vi "Image receiving and storage.vi"() -> ()   [LabVIEW 2009]
uses:
  <vilib>/vision/Image Controls.llb/IMAQ Image.ctl
panel:
  in  "A":bool=TRUE
  in  "¼v¹³Àx¦s¶s":bool
  in  "±i/¨C¬í":u32=30
  out "Àx¦s¸ô®|":path
  in  "connection in":string="dstp://192.168.1.100/image"
  in  "Äá¼v¾÷°±¤î¶s":bool
  out "«eÄá¼v¾÷":T1(plugin-control)
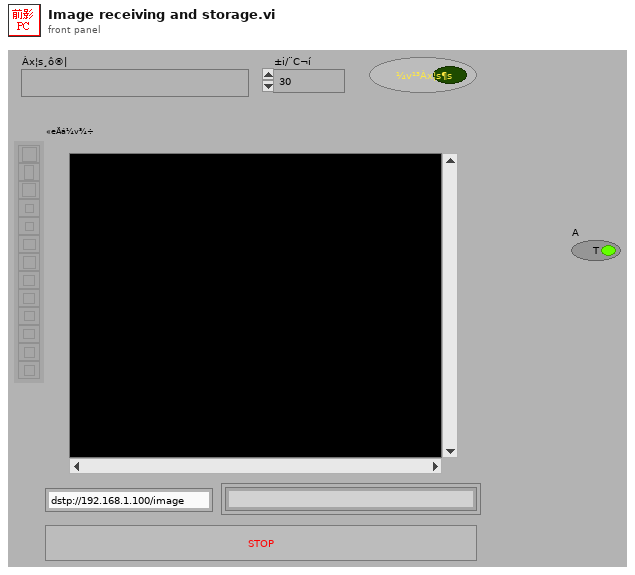
[diagram p1: front panel]
types:
  T1 = typedef "IMAQ Image.ctl" = refnum<image>
  T2 = enum16{"big-endian, network order", "native, host order", "little-endian"}
  T3 = enum32{"existing file", "new file", "new or existing file", "existing dir", "new dir", "new or existing dir", "existing file (use LLBs)", "new file (use LLBs)", "new or existing file (use LLBs)", "new or existing file or directory (use LLBs)"}
  T4 = typedef "AviRefnum.ctl" = refnum<k1>
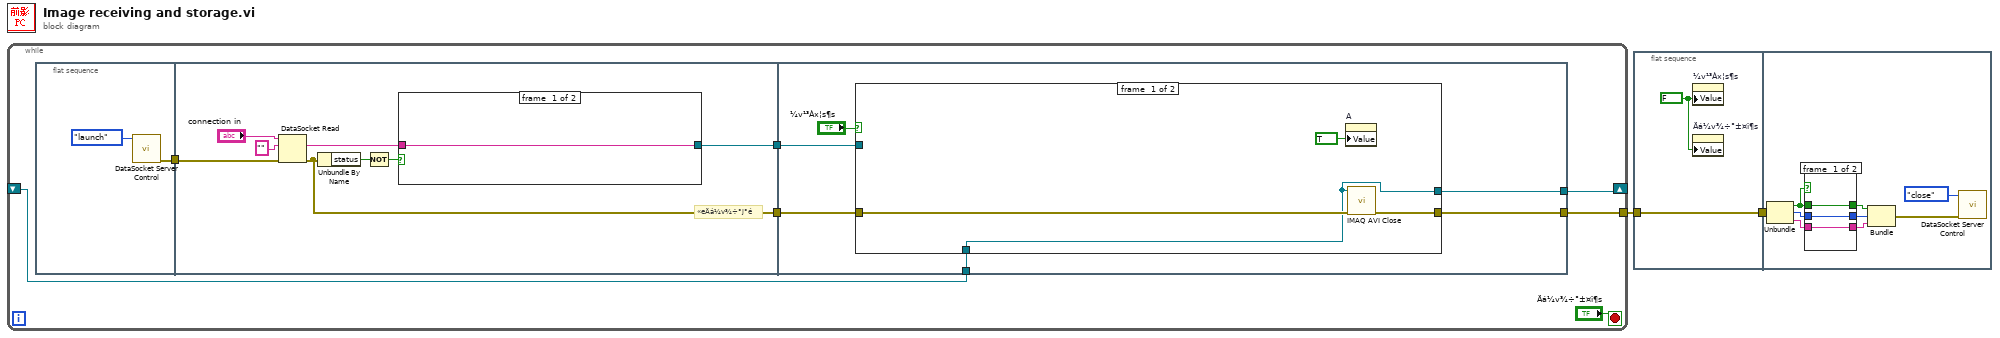
[diagram p0: block diagram]
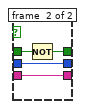
[diagram p2: hidden frame]
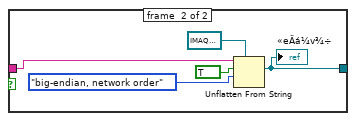
[diagram p3: hidden frame]
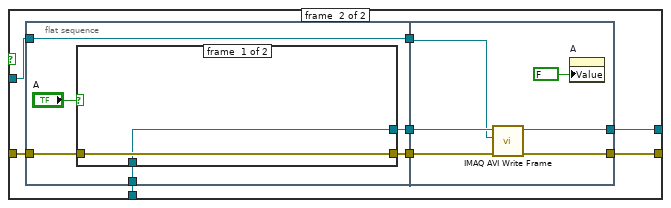
[diagram p4: hidden frame]
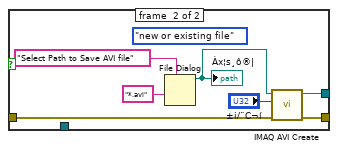
[diagram p5: hidden frame]
diagram:
  n1 = while {
    tunnel: [w6] -> w2
    shift-right: [w4] -> _
    shift-left: _ -> [w3]
    stop <- "Äá¼v¾÷°±¤î¶s" stop-if-true
    n2 = flat-sequence {
      tunnel: [w10] -> w9
      tunnel: w9 -> [w14]
      tunnel: [w13] -> w8
      tunnel: [w12] -> w5
      tunnel: w8 -> [w30]
      tunnel: w5 -> [w28]
      tunnel: [w29] -> w6
      tunnel: [w27] -> w4
      tunnel: w3 -> [w26]
      frame #0 {
        n3 = call <vilib>:"DataSocket Server Control.vi"("operation (launch)"=enum16{"launch", "show", "hide", "close"}."launch") -> ("error out"=w10:errorcluster)  [unwired: 1 in, 5 out]
      }
      frame #1 {
        # "«eÄá¼v¾÷°j°é"
        n4 = DataSocket Read(8:w14, 10:"", 11:"connection in") -> (0:w13:errorcluster, 2:w17:string)  [unwired: 7 out]
        n5 = Unbundle By Name(w13) -> ("status"=w15:bool)
        n6 = Not(x=w15) -> (.not. x?=w16:bool)
        n7 = case shown="False" w16 {
          tunnel: w17 -> [w20 w22]
          tunnel: [w20 w21] -> w12
          frame #0 {
          }
          frame #1 {
            n8 = Unflatten From String(type=T1 refnum ("Image"), binary string=w22, data includes array or string size? (T)=TRUE, byte order (0:big-endian, network order)=T2."big-endian, network order") -> (value=w21:T1)  [unwired: 1 in, 2 out]
            "«eÄá¼v¾÷" <- w21
          }
        }
      }
      frame #2 {
        n9 = case shown="True" "¼v¹³Àx¦s¶s" {
          tunnel: [w34 w39] -> w29
          tunnel: w30 -> [w35 w43]
          tunnel: w28 -> [_ w36]
          tunnel: [w33 w40] -> w27
          tunnel: w26 -> [w33 w38]
          frame #0 {
            n10 = property on="A" class="Bool (strict)"("Value"=TRUE ("A")) -> ()  [unwired: 2 in, 2 out]
            n11 = call "IMAQ AVI Close"("error in (no error)"=w35, "Avi Refnum"=w33) -> ("error out"=w34:errorcluster)  [unwired: 9 in]
          }
          frame #1 {
            n12 = flat-sequence {
              tunnel: w43 -> [w46]
              tunnel: [w48] -> w42
              tunnel: [w47] -> w41
              tunnel: w38 -> [w45]
              tunnel: [w44] -> w37
              tunnel: w36 -> [w44]
              tunnel: [w62] -> w39
              tunnel: w42 -> [w63]
              tunnel: w41 -> [w61]
              tunnel: [w60] -> w40
              tunnel: w37 -> [w59]
              frame #0 {
                n13 = case shown="True" "A" {
                  tunnel: w46 -> [w51 w54]
                  tunnel: [w51 w53] -> w48
                  tunnel: [w50 w52] -> w47
                  tunnel: w45 -> [w50 _]
                  frame #0 {
                  }
                  frame #1 {
                    (unwired) T3."new or existing file" ("select mode (2)")
                    n14 = File Dialog(7:"Select Path to Save AVI file" ("prompt"), 9:"*.avi" ("pattern")) -> (3:w57:path)  [unwired: 5 in, 3 out]
                    "Àx¦s¸ô®|" <- w57
                    n15 = call "IMAQ AVI Create"("error in (no error)"=w54, "Frames Per Second"="±i/¨C¬í", "AVI Path"=w57) -> ("error out"=w53:errorcluster, "Avi Refnum"=w52:T4)  [unwired: 7 in]
                  }
                }
              }
              frame #1 {
                n16 = call "IMAQ AVI Write Frame"("error in (no error)"=w63, "Image"=w59, "Avi Refnum"=w61) -> ("error out"=w62:errorcluster, "Avi Refnum (duplicate)"=w60:T4)  [unwired: 7 in]
                n17 = property on="A" class="Bool (strict)"("Value"=FALSE ("A")) -> ()  [unwired: 2 in, 2 out]
              }
            }
          }
        }
      }
    }
  }
  n18 = flat-sequence {
    tunnel: w2 -> [w65]
    tunnel: [w65] -> w1
    tunnel: w1 -> [w67]
    frame #0 {
      w66 = FALSE ("stop")
      n19 = property on="¼v¹³Àx¦s¶s" class="Bool (strict)"("Value"=w66) -> ()  [unwired: 2 in, 2 out]
      n20 = property on="Äá¼v¾÷°±¤î¶s" class="Bool (strict)"("Value"=w66) -> ()  [unwired: 2 in, 2 out]
    }
    frame #1 {
      n21 = Unbundle(w67) -> ("status"=w75:bool, "code"=w70:i32, "source"=w68:string)
      n22 = case shown="False" w75 {
        tunnel: [w76 w80] -> w72
        tunnel: [w78 w82] -> w71
        tunnel: w70 -> [w78 w82]
        tunnel: [w77 w81] -> w69
        tunnel: w68 -> [w77 w81]
        tunnel: w75 -> [w76 w79]
        frame #0 {
        }
        frame #1 {
          n23 = Not(x=w79) -> (.not. x?=w80:bool)
        }
      }
      n24 = Bundle("status"=w72, "code"=w71, "source"=w69) -> (w74:errorcluster)  [unwired: 1 in]
      n25 = call <vilib>:"DataSocket Server Control.vi"("error in (no error)"=w74, "operation (launch)"=enum16{"launch", "show", "hide", "close"}."close") -> ()  [unwired: 6 out]
    }
  }
